vi "DB_Eventos.vi"(8 "error in (no error)":errorcluster, 9 "Final":T1 format="%<%X\n%x>T", 10 "Inicio":T1 format="%<%X\n%x>T") -> (0 "error out":errorcluster, 3 "Data":string[][](array[string]))   [LabVIEW 2018]
uses:
  <vilib>/RAFA Solutions/Harmony UI Controls Kit/Numeric/Time Stamp Control.ctl
  <vilib>/addons/database/Connection.llb/DB Tools Open Connec (Path).vi
  <vilib>/addons/database/Connection.llb/Conn Execute.vi
  <vilib>/addons/database/Recordset.llb/Rec Fetch Recordset Data (R).vi
  <vilib>/addons/database/Recordset.llb/Rec Destroy - Connection.vi
  <vilib>/addons/database/_DB Variant To Data/Database Variant To Data.xnode
  <vilib>/addons/database/NI_Database_API.lvlib
  <vilib>/RAFA Solutions/Harmony UI Controls Kit/Flat UI Design.lvlib
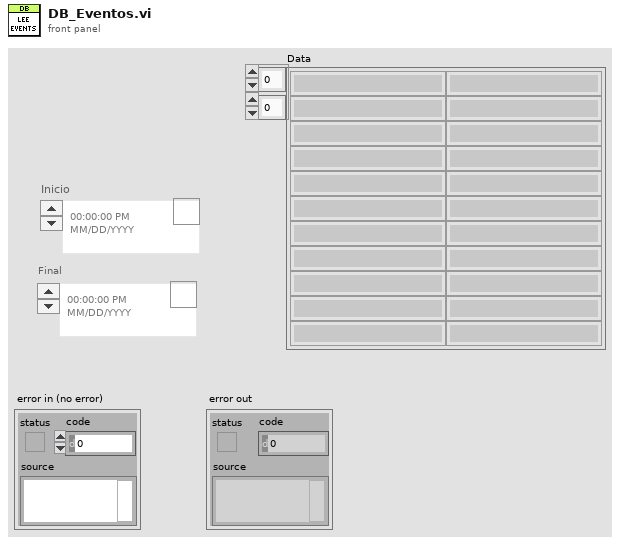
[diagram p1: front panel]
types:
  T1 = typedef "Flat UI Design.lvlib/Time Stamp Control.ctl" = timestamp
  T2 = typedef "NI_Database_API.lvlib/Conn ObjectReference.ctl" = refnum<k1>
  T3 = typedef "NI_Database_API.lvlib/Rec ObjectReference.ctl" = refnum<k1>
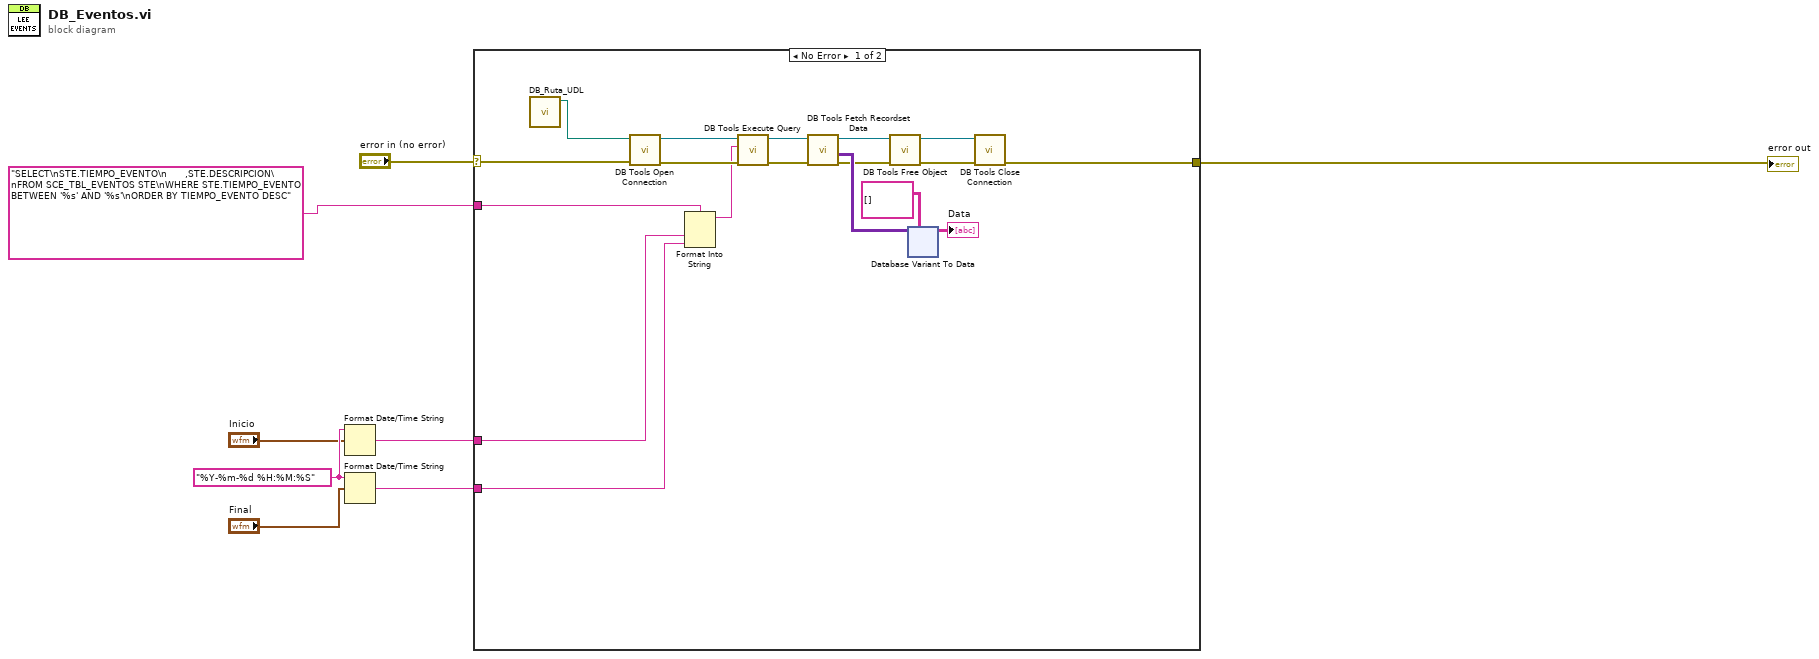
[diagram p0: block diagram]
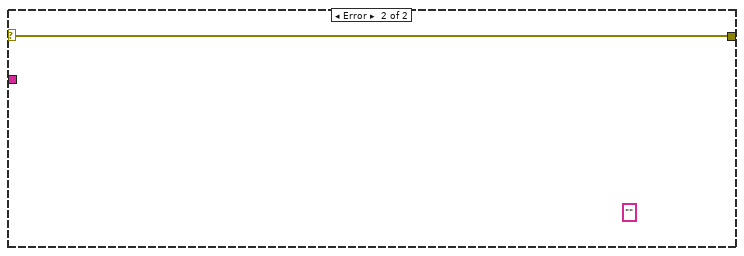
[diagram p2: hidden frame]
diagram:
  w5 = "%Y-%m-%d %H:%M:%S" ("time format string (%c)")
  n1 = Format Date/Time String(time format string (%c)=w5, seconds (now)="Inicio") -> (date/time string=w2:string)  [unwired: 1 in]
  n2 = Format Date/Time String(time format string (%c)=w5, seconds (now)="Final") -> (date/time string=w1:string)  [unwired: 1 in]
  n3 = case shown="No Error" "error in (no error)" {
    selector: "error in (no error)" -> [w21 w71]
    tunnel: [w23 w71] -> w7
    tunnel: "SELECT\nSTE.TIEMPO_EVENTO\n      ,STE.DESCRIPCION\nFROM SCE_TBL_EVENTOS STE\nWHERE STE.TIEMPO_EVENTO BETWEEN '%s' AND '%s'\nORDER BY TIEMPO_EVENTO DESC" ("SQL") -> [w14 _]
    tunnel: w2 -> [w12 _]
    tunnel: w1 -> [w11 _]
    frame No Error {
      n4 = call "DB_Ruta_UDL.vi"() -> ("UDL ruta"=w10:path)  [unwired: 11 in]
      n5 = call-poly <vilib>:"DB Tools Open Connection.vi"("error in (no error)"=w21, "connection information"=w10) -> ("error out"=w26:errorcluster, "connection reference"=w24:T2)  [unwired: 6 in]
      n6 = Format Into String(format string=w14, w12, w11) -> (resulting string=w13:string)  [unwired: 2 in, 1 out]
      n7 = call-poly <vilib>:"DB Tools Execute Query.vi"("error in (no error)"=w26, "SQL query"=w13, "connection reference"=w24) -> ("error out"=w22:errorcluster, "recordset reference"=w20:T3)  [unwired: 5 in]
      n8 = call-poly <vilib>:"DB Tools Fetch Recordset Data.vi"("error in (no error)"=w22, "recordset reference"=w20) -> ("error out"=w16:errorcluster, "recordset data"=w17:variant[][], "recordset reference out"=w19:T3)  [unwired: 3 in]
      n9 = call-poly <vilib>:"DB Tools Free Object.vi"("error in (no error)"=w16, "recordset reference"=w19) -> ("error out"=w25:errorcluster, "connection reference"=w9:T2)  [unwired: 8 in]
      n10 = xnode "Database Variant To Data"("database variant"=w17, "type"=string[][] []) -> ("data"=→"Data":string[][])  [unwired: 1 in, 1 out]
      n11 = call <vilib>:"DB Tools Close Connection.vi"("error in (no error)"=w25, "connection reference"=w9) -> ("error out"=w23:errorcluster)  [unwired: 5 in]
    }
    frame Error {
      (unwired) ""
    }
  }
  "error out" <- w7
